vi "ClusterRefFromPath.vi"(8 "error in":errorcluster, 10 "Cluster Path":path) -> (0 "error out":errorcluster, 2 "Cluster.ctl ref":refnum<vi>, 3 "Ref cluster":T1)   [LabVIEW 2025, in "UI_Library.lvlib" / "UI_Library.lvclass"]
doc: "Obtain the references of all the controls of the Cluster data"
uses:
  UI_Library.lvclass
  Controls/UI_RefCluster.ctl
  <vilib>/Utility/Data Type/Type Definitions/Data Type.ctl
  <vilib>/Utility/Data Type/NI_Data Type.lvlib
  UI_Library.lvlib
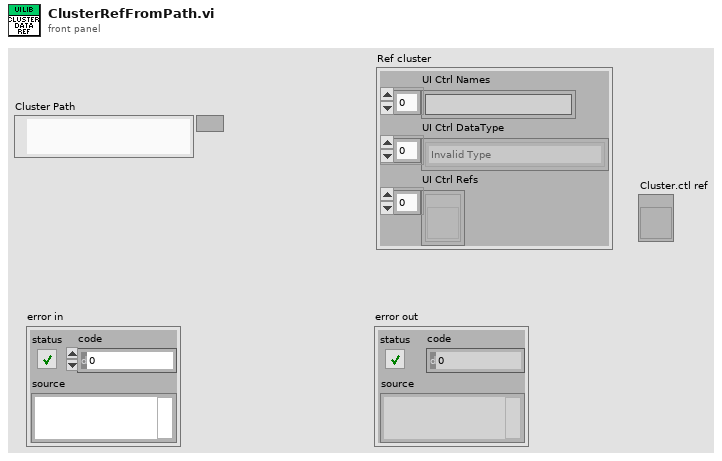
[diagram p1: front panel]
types:
  T1 = typedef "UI_Library.lvlib/UI_RefCluster.ctl" = cluster{"UI Ctrl Names":string[], "UI Ctrl DataType":T2[], "UI Ctrl Refs":refnum<vi>[]}
  T2 = typedef "NI_Data Type.lvlib/Data Type.ctl" = enum8{"Invalid Type", "Void", "I8", "I16", "I32", "I64", "U8", "U16", "U32", "U64", "Single Float", "Double Float", "Extended Float", "Single Complex", "Double Complex", "Extended Complex", "Enum U8", "Enum U16", "Enum U32", "Enum U64", "Single Float With Unit", "Double Float With Unit", "Extended Float With Unit", "Single Complex with Unit", "Double Complex with Unit", "Extended Complex with Unit", "Boolean", "String", "Path", "Picture", "Tag", "Array", "Cluster", "Variant", "LV Variant", "Waveform", "Timestamp", "Digital Waveform", "Digital Data", "ExpressData", "Refnum", "External Data", "VI", "Poly VI", "LabVIEW Class Instance", "Fixed Point", "Set Collection", "Map Collection"}
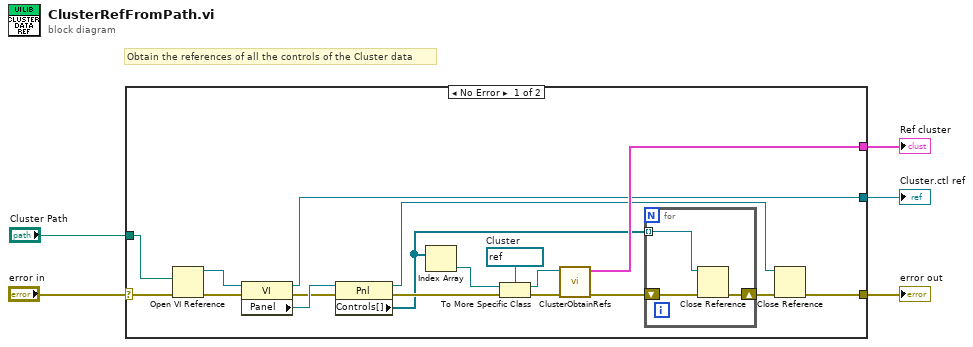
[diagram p0: block diagram]
diagram:
  # "Obtain the references of all the controls of the Cluster data"
  n1 = case shown="No Error" "error in" {
    selector: "error in" -> [w16 w27]
    tunnel: "Cluster Path" -> [w22 _]
    tunnel: [w17 _] -> w4
    tunnel: [w8 w27] -> w2
    tunnel: [w6 _] -> w1
    frame No Error {
      w18 = refnum<vi> refnum  # Cluster
      n2 = Open VI Reference(vi path=w22, error in (no error)=w16) -> (vi reference=w21:refnum<vi>, error out=w15:errorcluster)  [unwired: 4 in]
      n3 = property on="Property Node" class="VI"(reference=w21, error in=w15) -> (reference out=w6:refnum<vi>, error out=w13:errorcluster, "Panel"=w23:refnum<vi>)
      n4 = property on="Property Node" class="Pnl"(reference=w23, error in=w13) -> (reference out=w7:refnum<vi>, error out=w12:errorcluster, "Controls[]"=w10:refnum<vi>[])
      n5 = Index Array(array=w10) -> (element=w20:refnum<vi>)  [unwired: 1 in]
      n6 = To More Specific Class(target class=w18, reference=w20, error in=w12) -> (specific class reference=w19:refnum<vi>, error out=w14:errorcluster)
      n7 = call "ClusterObtainRefs.vi"("error in (no error)"=w14, "Clust Refnum"=w19) -> ("error out"=w11:errorcluster, "Ref cluster"=w17:T1)  [unwired: 8 in]
      n8 = for {
        shift-right: [w25] -> w9
        shift-left: w11 -> [w26]
        tunnel: w10 -> [w24] mode=indexing
        n9 = Close Reference(reference=w24, error in (no error)=w26) -> (error out=w25:errorcluster)
      }
      n10 = Close Reference(reference=w7, error in (no error)=w9) -> (error out=w8:errorcluster)
    }
    frame Error {
    }
  }
  "Ref cluster" <- w4
  "error out" <- w2
  "Cluster.ctl ref" <- w1
